vi "SavingFPtoINIfile.vi"() -> ()   [LabVIEW 2021]
panel:
  in  "myArray":cluster{"Numeric":dbl, "String":string}[](array[cluster])=[{"Numeric"=0.0, "String"="zero"}, {"Numeric"=1.0, "String"="one"}, {"Numeric"=2.0, "String"="two"}]
  in  "cantSaveLatches":bool
  in  "Cluster":cluster{"Numeric":dbl, "String":string}
  in  "Mode":enum16{"Read", "Write"}(ring)=enum."Write"
  in  "OK Button":bool
  out "LEDindicator":bool
  in  "aPath":path
  in  "Tab Control":enum32{"Page 1", "Page 2", "Page 3"}(tab)
  in  "String 2":string
  in  "Enum":enum16{"enum val 0", "enum val1"}(ring)
  in  "Combo Box":string(combo)
  in  "Tab Control 2":enum32{"Page 1", "Page 2"}(tab)
  in  "Checkbox":bool
  in  "Numeric 2":dbl
  # "Example of how to save/ load all FP values to/from and INI file.\n\nHow to use:\n\nSet up some values on the FP- add additional controls if desired\nSet Mode to \"Write\" and run VI.\n-Create a new file to save values to when prompted\n\nChange FP values, add/ remove controls\nSet Mode to \"Read\", run VI, and point to saved file\n-Everything gets put back to how it was saved!"
  # "For the array to save magically, you must only have a single element visible- so you can have a hidden copy with just a single element visible"
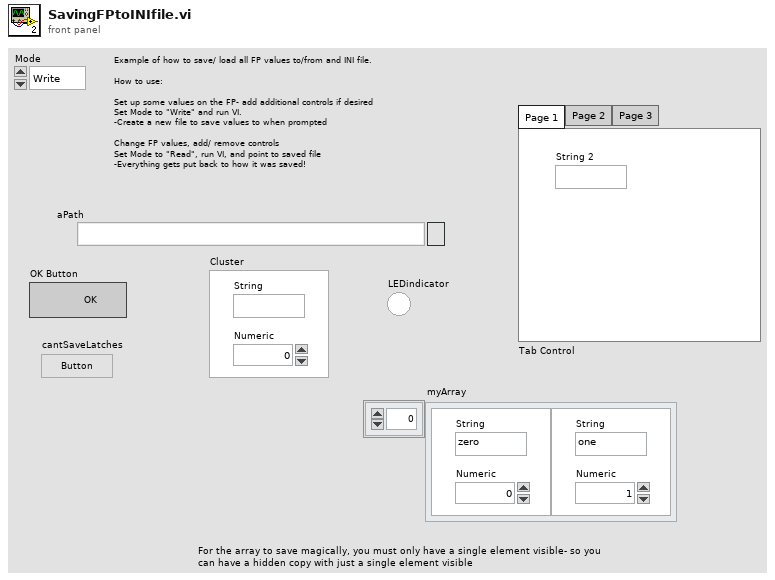
[diagram p1: front panel]
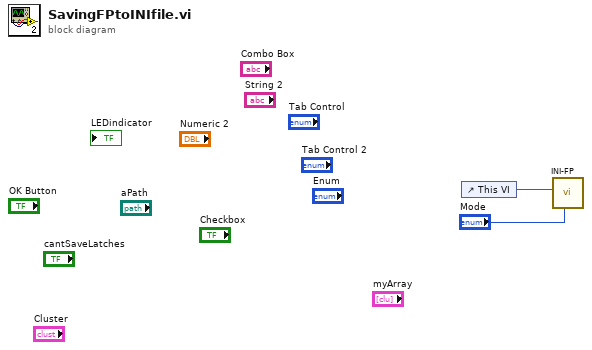
[diagram p0: block diagram]
diagram:
  n1 = control-ref of="This VI"() -> (w1:refnum<vi>)
  n2 = call "INI-FP.vi"("Mode"="Mode", "VIreference"=w1) -> ()  [unwired: 8 in, 2 out]
